vi "Agilent 3352X Series Software Triggered Frequency Sweep.vi"() -> ()   [LabVIEW 2015]
doc: "This example shows how to configure and enable a triggered frequency sweep."
uses:
  <instrlib>/Agilent 3352X Series/Agilent 3352X Series.lvlib
panel:
  in  "Start Frequency (100 Hz)":dbl=100.0
  in  "Sweep Time (1 s)":dbl=1.0
  in  "Stop  Frequency (1000 Hz)":dbl=1000.0
  in  "Waveform Function (0: Sine)":u16(ring) items=["Sine"=0, "Square"=1, "Ramp"=2, "Noise"=3, "DC"=4, "Triangle"=5, "Pulse"=6, "Sinc"=11, "D-Lorentz"=12, "Gaussian"=13, "Expo Fall"=14, "Expo Rise"=15, "Haversine"=16]
  in  "Amplitude (0.1 Vpp)":dbl=0.1
  in  "VISA resource name":refnum<visa-resource-name>
  # "(c) 2011-2015 National Instruments.  ALL RIGHTS RESERVED."
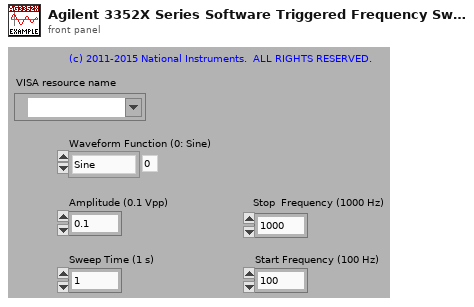
[diagram p1: front panel]
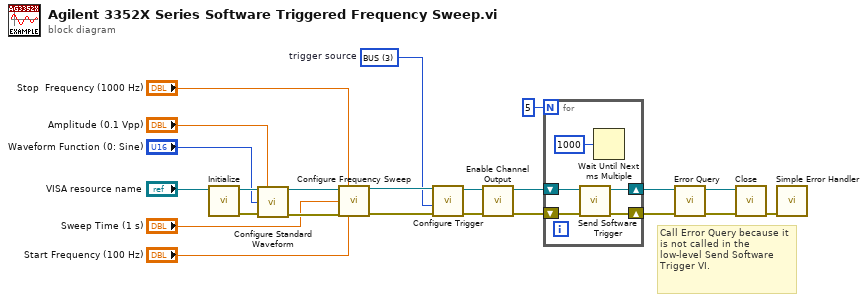
[diagram p0: block diagram]
diagram:
  w10 = 3 items=["IMMediate", "EXTernal", "TIMer", "BUS"]  # trigger source
  # "Call Error Query because it is not called in the low-level Send Software Trigger VI."
  n1 = call <instrlib>:"Initialize.vi"("VISA resource name"="VISA resource name") -> ("error out"=w8:errorcluster, "VISA resource name out"=w9:refnum<visa-resource-name>)  [unwired: 4 in, 5 out]
  n2 = call <instrlib>:"Configure Standard Waveform.vi"("VISA resource name"=w9, "Amplitude (0.1 Vpp)"="Amplitude (0.1 Vpp)", "Waveform Function (0: Sine)"="Waveform Function (0: Sine)", "error in (no error)"=w8) -> ("VISA resource name out"=w7:refnum<visa-resource-name>, "error out"=w6:errorcluster)  [unwired: 6 in, 4 out]
  n3 = call <instrlib>:"Configure Frequency Sweep.vi"("VISA resource name"=w7, "Stop  Frequency (1000 Hz)"="Stop  Frequency (1000 Hz)", "Sweep Time (1 s)"="Sweep Time (1 s)", "error in (no error)"=w6, "Start Frequency (100 Hz)"="Start Frequency (100 Hz)") -> ("VISA resource name out"=w12:refnum<visa-resource-name>, "error out"=w11:errorcluster)  [unwired: 4 in, 5 out]
  n4 = call <instrlib>:"Configure Trigger.vi"("error in (no error)"=w11, "Trigger Source (0: Immediate)"=w10, "VISA resource name"=w12) -> ("error out"=w21:errorcluster, "VISA resource name out"=w20:refnum<visa-resource-name>)  [unwired: 5 in, 2 out]
  n5 = call <instrlib>:"Enable Channel Output.vi"("error in (no error)"=w21, "VISA resource name"=w20) -> ("error out"=w17:errorcluster, "VISA resource name out"=w19:refnum<visa-resource-name>)  [unwired: 3 in, 5 out]
  n6 = for {
    N: 5 -> [_]
    shift-right: [w26] -> w14
    shift-left: w17 -> [w24]
    shift-right: [w27] -> w16
    shift-left: w19 -> [w28]
    n7 = call <instrlib>:"Send Software Trigger.vi"("error in (no error)"=w24, "VISA resource name"=w28) -> ("error out"=w26:errorcluster, "VISA resource name out"=w27:refnum<visa-resource-name>)  [unwired: 8 out]
    n8 = Wait Until Next ms Multiple(millisecond multiple=u32 1000) -> ()  [unwired: 1 out]
  }
  n9 = call <instrlib>:"Error Query.vi"("error in (no error)"=w14, "VISA resource name"=w16) -> ("error out"=w13:errorcluster, "VISA resource name out"=w15:refnum<visa-resource-name>)  [unwired: 8 out]
  n10 = call <instrlib>:"Close.vi"("error in (no error)"=w13, "VISA resource name"=w15) -> ("error out"=w23:errorcluster)  [unwired: 9 out]
  n11 = call <vilib>:"Simple Error Handler.vi"("error in (no error)"=w23) -> ()  [unwired: 1 in, 8 out]
